vi "CRYPEAQ RFFTMSq.vi"(10 "N":dbl, 11 "X":dbl[](array[numeric]) format="%#.6f") -> (3 "X2":dbl[](array[numeric]))   [LabVIEW 2013]
panel:
  # "Error Value = 0.00307786"
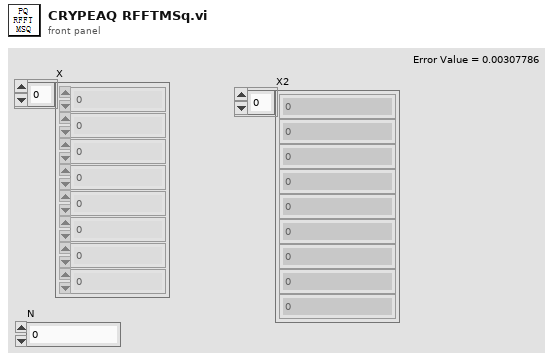
[diagram p1: front panel]
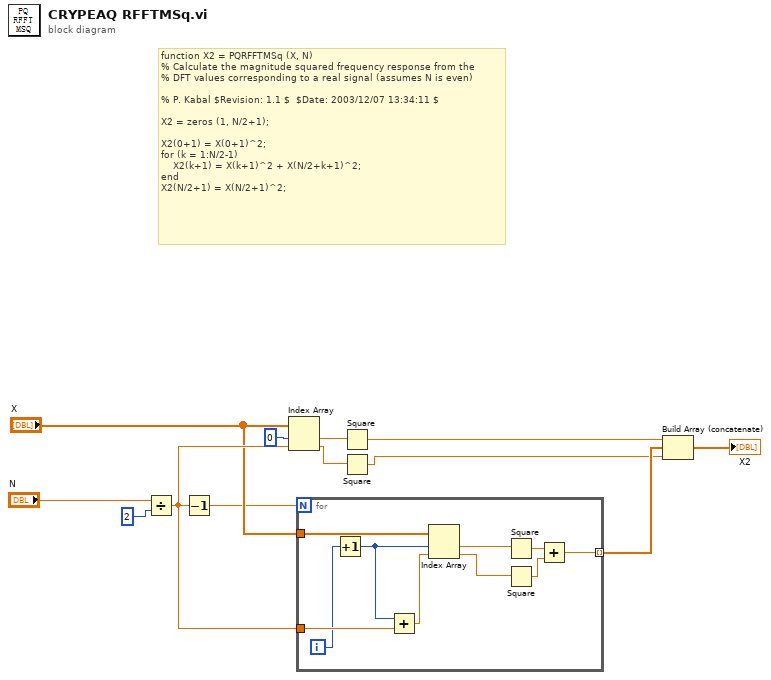
[diagram p0: block diagram]
diagram:
  # "function X2 = PQRFFTMSq (X, N)\n% Calculate the magnitude squared frequency response from the\n% DFT values corresponding to a real signal (assumes N is even)\n\n% P. Kabal $Revision: 1.1 $  $Date: 2003/12/07 13:34:11 $\n\nX2 = zeros (1, N/2+1);\n\nX2(0+1) = X(0+1)^2;\nfor (k = 1:N/2-1)\n    X2(k+1) = X(k+1)^2 + X(N/2+k+1)^2;\nend\nX2(N/2+1) = X(N/2+1)^2;"
  n1 = Divide(x="N", y=2) -> (x/y=w9:dbl)
  n2 = Decrement(x=w9) -> (x-1=w6:dbl)
  n3 = Index Array(array="X", index #1=0 ("index"), index #2=w9) -> (element #1=w2:dbl, element #2=w4:dbl)
  n4 = for {
    N: w6 -> [_]
    tunnel: "X" -> [w19]
    tunnel: w9 -> [w22]
    tunnel: [w20] -> w7 mode=indexing
    i -> [w21]
    n5 = Increment(x=w21) -> (x+1=w18:i32)
    n6 = Add(x=w18, y=w22) -> (x+y=w17:dbl)
    n7 = Index Array(array=w19, index #1=w18, index #2=w17) -> (element #1=w15:dbl, element #2=w16:dbl)
    n8 = Square(x=w15) -> (x^2=w14:dbl)
    n9 = Square(x=w16) -> (x^2=w13:dbl)
    n10 = Add(x=w14, y=w13) -> (x+y=w20:dbl)
  }
  n11 = Square(x=w2) -> (x^2=w1:dbl)
  n12 = Square(x=w4) -> (x^2=w3:dbl)
  n13 = Build Array (concatenate)(w1, w7, w3) -> (→"X2":dbl[])
